vi "Passwortlevel aendern.vi"(8 "geforderter Level":i16, 10 "Passworte":T3=[{"Name"="123", "Passwort"="", "Level"=0}, {"Name"="otto", "Passwort"="", "Level"=0}, {"Name"="iag", "Passwort"="", "Level"=0}], 11 "aktueller Level":i16) -> (0 "Freigabe":bool, 3 "aktueller Level":i16)   [LabVIEW 2020, in "Passwort.lvlib"]
uses:
  Passwort.lvlib
  Visualisierungs Elemente/String - Eingabefeld.ctl
  Passwort Array.ctl
  Visualisierungs Elemente/Button.ctl
  Visualisierungs Elemente/Zahlen-Ausgabefeld.ctl
  Sprachverwaltung/FGV Aktion Tabelle zerlegen.ctl
  SysLog/SysLog Interface.ctl
  Sprachverwaltung/Sprachverwaltung.lvlib
  SysLog/SysLog.lvlib
panel:
  out "Aktueller Level":T1
  in  "abbrechen":T2
  in  "Passwort":T4
  # "Der aktuelle Passwort-Level erlaubt den Zugriff nicht.\nGeben Sie Ihr Passwort ein:"
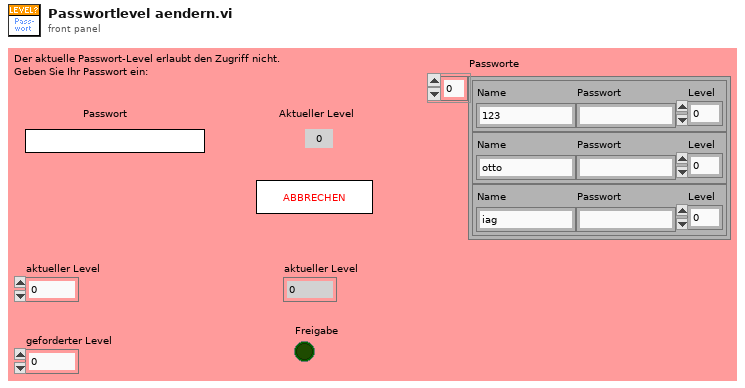
[diagram p1: front panel]
types:
  T1 = typedef "Zahlen-Ausgabefeld.ctl" = sgl
  T2 = typedef "Button.ctl" = bool
  T3 = typedef "Passwort.lvlib/Passwort Array.ctl" = cluster{"Name":string, "Passwort":string, "Level":i16}[]
  T4 = typedef "String - Eingabefeld.ctl" = string
  T5 = typedef "Sprachverwaltung.lvlib/FGV Aktion Tabelle zerlegen.ctl" = enum16{"laden", "vereinzeln", "speichern"}
  T6 = typedef "SysLog.lvlib/SysLog Interface.ctl" = cluster{"FehlermeldungsCode":i32, "ErfolgsmeldungsCode":i32, "ParameterListenString":string, "Anzeige":bool, "SysLogIcon":enum16{"OK", "Warnung", "Fehler"}, "intern":bool}
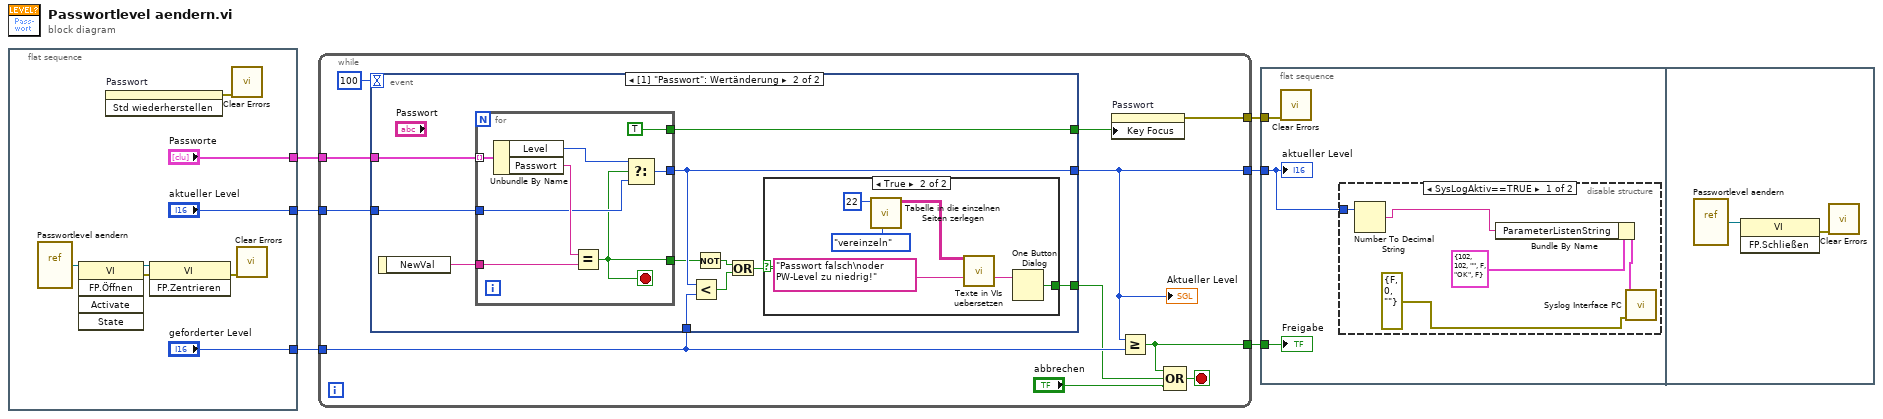
[diagram p0: block diagram]
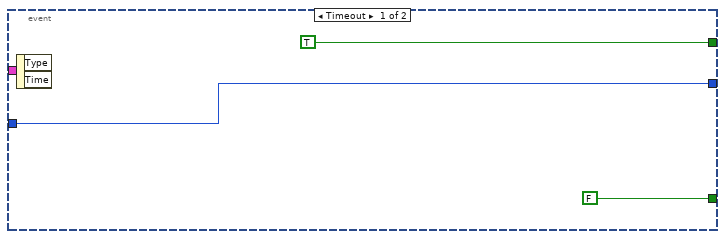
[diagram p3: hidden frame]
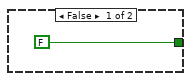
[diagram p4: hidden frame]
diagram:
  n1 = flat-sequence {
    tunnel: ["aktueller Level"] -> w6
    tunnel: ["geforderter Level"] -> w3
    tunnel: ["Passworte"] -> w2
    frame #0 {
      n2 = vi-ref "Passwortlevel aendern.vi"() -> (w9:refnum<vi>)
      n3 = invoke class="VI" method="FP.Öffnen"(reference=w9) -> (reference out=w8:refnum<vi>, error out=w7:errorcluster)  [unwired: 4 in, 3 out]
      n4 = invoke on="Passwort" class="Str (strikt)" method="Std wiederherstellen"() -> (error out=w11:errorcluster)  [unwired: 3 in, 2 out]
      n5 = invoke class="VI" method="FP.Zentrieren"(reference=w8, error in=w7) -> (error out=w10:errorcluster)  [unwired: 1 in, 2 out]
      n6 = call <vilib>:"Clear Errors.vi"("error in (no error)"=w11) -> ()  [unwired: 5 in, 2 out]
      n7 = call <vilib>:"Clear Errors.vi"("error in (no error)"=w10) -> ()  [unwired: 5 in, 2 out]
    }
  }
  n8 = while {
    tunnel: w6 -> [w25]
    tunnel: [w23] -> w5
    tunnel: [w18] -> w4
    tunnel: w3 -> [w20]
    tunnel: w2 -> [w22]
    tunnel: [w15] -> w1
    stop <- w16 stop-if-true
    n9 = event shown="[1] \"Passwort\": Wertänderung" {
      selector: _ -> [_ _]
      dyn-events: _ -> [_ _]
      timeout: 100 -> [_ _]
      tunnel: w25 -> [w27 w39]
      tunnel: [TRUE ("Tastaturfokus") w38] -> w24
      tunnel: [w27 w34] -> w23
      tunnel: w22 -> [_ w37]
      tunnel: w20 -> [_ w33]
      tunnel: [FALSE ("true") w31] -> w17
      event Timeout {
        n10 = event-data() -> ()  [unwired: 1 in, 2 out]
      }
      event Value Change {
        n11 = event-data() -> ("NewVal"=w36:T4)  [unwired: 1 in]
        n12 = for {
          tunnel: w36 -> [w53]
          tunnel: w37 -> [w54] mode=indexing
          tunnel: w39 -> [w50]
          tunnel: [w49] -> w34
          tunnel: [TRUE ("Tastaturfokus")] -> w38
          tunnel: [w47] -> w29
          stop <- w47 stop-if-true
          n13 = Unbundle By Name(w54) -> ("Level"=w51:i16, "Passwort"=w52:string)
          n14 = Equal?(x=w52, y=w53) -> (x = y?=w47:bool)
          n15 = Select(t=w51, s=w47, f=w50) -> (s? t:f=w49:i16)
        }
        n16 = Less?(x=w34, y=w33) -> (x < y?=w35:bool)
        n17 = Not(x=w29) -> (.not. x?=w30:bool)
        n18 = Or(x=w30, y=w35) -> (x .or. y?=w32:bool)
        n19 = case shown="True" w32 {
          tunnel: [FALSE ("true") w46] -> w31
          frame False {
          }
          frame True {
            n20 = call "Tabelle in die einzelnen Seiten zerlegen.vi"("Aktion"=FGV_Aktion_Tabelle_zerlegen."vereinzeln", "Index (Seite)"=22) -> ("Sprachliste"=w42:string[][])  [unwired: 7 in, 2 out]
            n21 = call "Texte in VIs uebersetzen.vi"("Sprachliste"=w42, "String zum Übersetzen"="Passwort falsch\noder PW-Level zu niedrig!" ("Nachricht")) -> ("String zum Übersetzen"=w44:string)  [unwired: 9 in, 4 out]
            n22 = One Button Dialog(message=w44) -> (true=w46:bool)  [unwired: 1 in]
          }
        }
      }
    }
    "Aktueller Level" <- w23
    n23 = property on="Passwort" class="Str (strikt)"("Key Focus"=w24) -> (error out=w15:errorcluster)  [unwired: 2 in, 1 out]
    n24 = Greater Or Equal?(x=w23, y=w20) -> (x >= y?=w18:bool)
    n25 = Compound Arithmetic op=OR(w18, w17, "abbrechen") -> (w16:T2)
  }
  n26 = flat-sequence {
    tunnel: w5 -> [w55]
    tunnel: w4 -> [w57]
    tunnel: w1 -> [w56]
    frame #0 {
      n27 = call <vilib>:"Clear Errors.vi"("error in (no error)"=w56) -> ()  [unwired: 5 in, 2 out]
      n28 = disable-structure shown="SysLogAktiv==TRUE" {
        disable-tunnel: w55 -> [w62 _]
        frame condition #0 (active) {
          n29 = Number To Decimal String(number=w62) -> (decimal integer string=w58:string)  [unwired: 1 in]
          n30 = Bundle By Name(cluster=T6 {"FehlermeldungsCode"=102, "ErfolgsmeldungsCode"=102, "ParameterListenString"="", "Anzeige"=FALSE, "SysLogIcon"=enum."OK", "intern"=FALSE} ("Cluster (in)"), "ParameterListenString"=w58) -> (w59:T6)
          n31 = call "Syslog Interface PC.vi"("Fehler (in)"=errorcluster {"status"=FALSE, "code"=0, "source"=""}, "Cluster (in)"=w59) -> ()  [unwired: 9 in, 1 out]
        }
        frame condition #1 {
        }
      }
      "aktueller Level" <- w55
      "Freigabe" <- w57
    }
    frame #1 {
      n32 = vi-ref "Passwortlevel aendern.vi"() -> (w64:refnum<vi>)
      n33 = invoke class="VI" method="FP.Schließen"(reference=w64) -> (error out=w63:errorcluster)  [unwired: 2 in, 2 out]
      n34 = call <vilib>:"Clear Errors.vi"("error in (no error)"=w63) -> ()  [unwired: 5 in, 2 out]
    }
  }
